vi "Kernel Workgroup Information.vi"(8 "Error In":errorcluster, 9 "Kernel Handle":T2, 11 "Device ID":T3) -> (0 "Error Out":errorcluster, 1 "Kernel Handle":T2, 3 "Device ID":T3, 4 "Kernel Information":T1)   [LabVIEW 2012]
doc: "This VI returns information about a kernel that is required if the <b>Execute Kernel Advanced</b> function is going to be used with Workgroup information. Information such as Workgroup Size, Workgroup Multiple, and kernel memory information can be found here."
uses:
  Non-User VIs/Controls/Device ID.ctl
  Non-User VIs/Controls/Kernel Handle.ctl
  Non-User VIs/Controls/Kernel Workgroup Information.ctl
  Non-User VIs/Error Checking/Add Error Functional Global.vi
  OpenCLV x64.lvlib
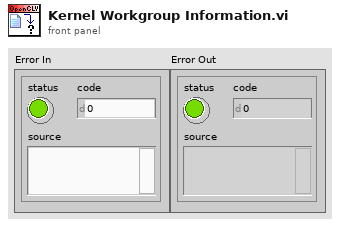
[diagram p1: front panel]
types:
  T1 = typedef "OpenCLV x64.lvlib/Kernel Workgroup Information.ctl" = cluster{"Compile Workgroup Size":u64[], "Kernel Private Mem":u64, "Kernel Local Mem":u64, "Work Group Multiple":u64, "Max Work Group Size":u64}
  T2 = typedef "OpenCLV x64.lvlib/Kernel Handle.ctl" = u64
  T3 = typedef "OpenCLV x64.lvlib/Device ID.ctl" = u64
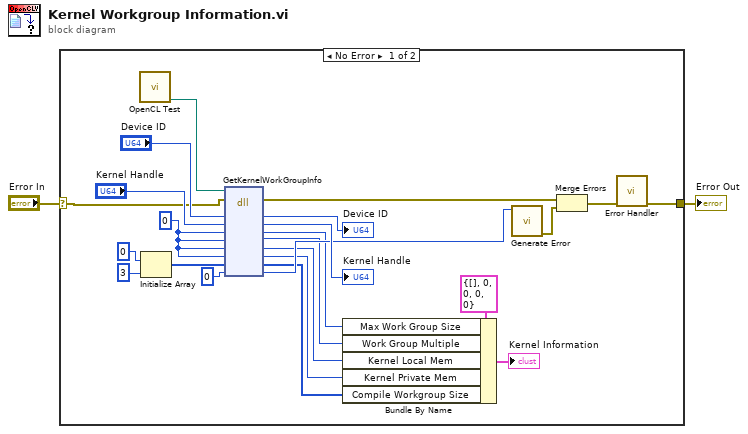
[diagram p0: block diagram]
diagram:
  n1 = case shown="No Error" "Error In" {
    selector: "Error In" -> [w3 w26]
    tunnel: [w7 w26] -> w1
    frame No Error {
      w16 = u64 0 ("Kernel Private Mem")
      n2 = call "OpenCL Test.vi"() -> ("DLL To Use"=w8:path)  [unwired: 11 in]
      n3 = Initialize Array(u64 0 ("element"), 3 ("dimension size")) -> (w22:u64[])
      n4 = dll-call lib="C:/Users/bme-amcelroy-la/Desktop/OpenCLV/trunk/OpenCLV_x64_1.0/OpenCLV_x64.dll" fn="GetKernelWorkGroupInfo"(path in=w8, error in=w3, "Labview Device"="Device ID", "Kernel Handle"="Kernel Handle", "Max Workgroup Size"=w16, "Workgroup Multiple"=w16, "Kernel Local Mem"=w16, "Kernel Private Mem"=w16, "Compile Workgroup Size"=w22, "Error"=0) -> (error out=w4:errorcluster, "Labview Device"=→"Device ID":u64, "Kernel Handle"=→"Kernel Handle":u64, "Max Workgroup Size"=w14:u64, "Workgroup Multiple"=w13:u64, "Kernel Local Mem"=w12:u64, "Kernel Private Mem"=w11:u64, "Compile Workgroup Size"=w10:u64[], "Error"=w17:i32)  [unwired: 2 in, 1 out]
      n5 = Bundle By Name(cluster=T1 {"Compile Workgroup Size"=[], "Kernel Private Mem"=0, "Kernel Local Mem"=0, "Work Group Multiple"=0, "Max Work Group Size"=0} ("Kernel Information 2"), "Max Work Group Size"=w14, "Work Group Multiple"=w13, "Kernel Local Mem"=w12, "Kernel Private Mem"=w11, "Compile Workgroup Size"=w10) -> (→"Kernel Information":T1)
      n6 = call "Generate Error.vi"("Error"=w17) -> ("error out"=w6:errorcluster)  [unwired: 10 in]
      n7 = Merge Errors(w4, w6) -> (w5:errorcluster)
      n8 = call-poly "Error Handler.vi"("Error In"=w5) -> ("Error Out"=w7:errorcluster)  [unwired: 10 in]
    }
    frame Error {
    }
  }
  "Error Out" <- w1
